vi "TempControlLogica.vi"(1 "setwaarde":string, 3 "input":string) -> (9 "output":string, 11 "temp grooter dan setwaardde":bool)   [LabVIEW 2013]
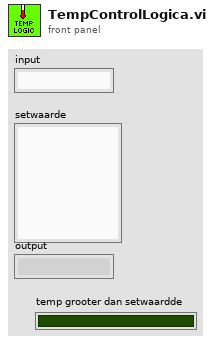
[diagram p1: front panel]
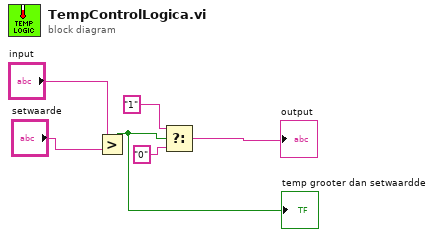
[diagram p0: block diagram]
diagram:
  n1 = Greater?(x="input", y="setwaarde") -> (0:w1:bool)
  "temp grooter dan setwaardde" <- w1
  n2 = Select(t="1", s=w1, f="0") -> (s? t:f=→"output":string)
